vi "onTerminateSession.vi"(8 "error in (no error)":errorcluster, 10 "Destroy (T)":bool=TRUE, 11 "Session.Server in":refnum<class "Session.Server.lvclass">) -> (0 "error out":errorcluster, 2 "Session Destroyed":bool, 3 "Session.Server out":refnum<class "Session.Server.lvclass">)   [LabVIEW 2013, in "MQTT Server.lvlib" / "Session.Server.lvclass"]
uses:
  Session.Server.lvclass
  MQTT_Base/Session/Session.lvclass
  MQTT_Base/Session/Session.lvclass/Session.ctl
  StoredSessions/StoredSessions.lvclass
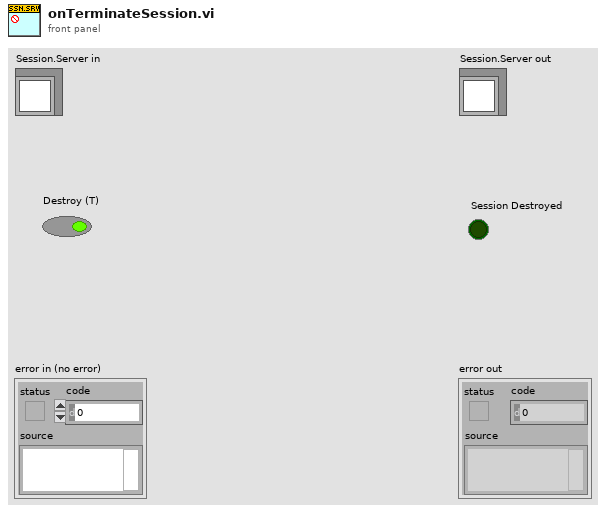
[diagram p1: front panel]
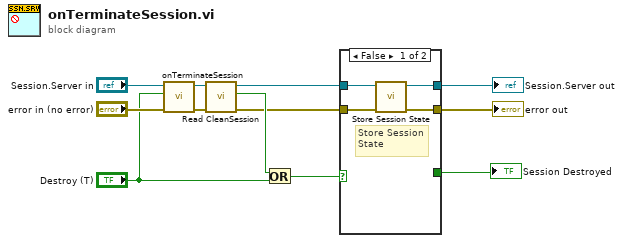
[diagram p0: block diagram]
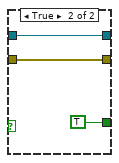
[diagram p2: hidden frame]
diagram:
  n1 = call-parent "onTerminateSession.vi"("error in (no error)"="error in (no error)", "Destroy (T)"="Destroy (T)", "Session in"="Session.Server in") -> ("error out"=w7:errorcluster, "Session out"=w8:refnum<class "Session.Server.lvclass">)  [unwired: 6 in, 1 out]
  n2 = call "Read CleanSession.vi"("error in (no error)"=w7, "Session in"=w8) -> ("error out"=w3:errorcluster, "CleanSession"=w10:bool, "Session out"=w6:refnum<class "Session.Server.lvclass">)  [unwired: 7 in]
  n3 = Or(x=w10, y="Destroy (T)") -> (x .or. y?=w4:bool)
  n4 = case shown="False" w4 {
    tunnel: [w15 w18] -> w2
    tunnel: [_ TRUE] -> w1
    tunnel: w3 -> [w16 w18]
    tunnel: [w13 w17] -> w5
    tunnel: w6 -> [w14 w17]
    frame False {
      # "Store Session\nState"
      n5 = call "Store Session State.vi"("error in (no error)"=w16, "Session"=w14) -> ("error out"=w15:errorcluster, "Session dup"=w13:refnum<class "Session.Server.lvclass">)  [unwired: 8 in]
    }
    frame True {
    }
  }
  "error out" <- w2
  "Session.Server out" <- w5
  "Session Destroyed" <- w1
